vi "GetStatusGenericDrive.vi"(0 "Channel Properties":T1={"Channel Name"="", "Vel. Default"=5.0, "Acc. Default"=5.0, "Vel. Max"=5.0, "Vel. Min"=5.0, "Acc. Max"=5.0, "Acc. Min"=5.0, "Pulses/unit"=0.0, "Address"=0, "Pulse Offset"=0, "Pos Tolerance"=0.0, "Pulses/rev"=0.0, "Backlash/Eng units"=0.0, "Current Pos"=0.0, "Ch Status"=enum."Active", "Port Name"="", "Axis Transform mode"="", "Metadata Ch Name"="", "Type"=""} {"Current Pos" format="%.2f"; "Backlash/Eng units" format="%.2f"; "Pulses/rev" format="%.2f"; "Pos Tolerance" format="%.2f"; "Pulses/unit" format="%.2f"; "Acc. Min" format="%.2f"; "Acc. Max" format="%.2f"; "Vel. Min" format="%.2f"; "Vel. Max" format="%.2f"; "Acc. Default" format="%.2f"; "Vel. Default" format="%.2f"}, 2 "Limit switch valid?":bool, 3 "Stop on Trigger 3?":bool) -> (5 "Ready":bool, 6 "OK":bool, 7 "Position in Move":dbl format="%.2f", 8 "Error string":string)   [LabVIEW 2010]
uses:
  DriveProperties.ctl
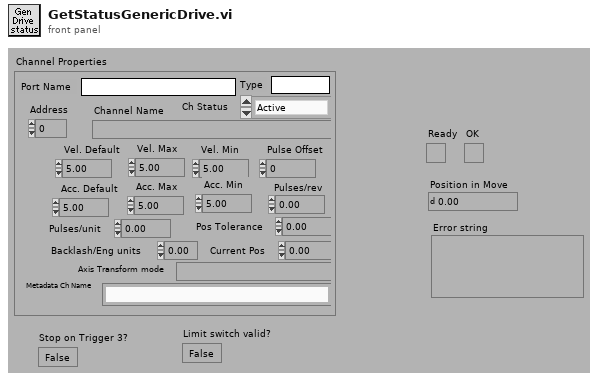
[diagram p1: front panel]
types:
  T1 = typedef "DriveProperties.ctl" = cluster{"Channel Name":string, "Vel. Default":dbl, "Acc. Default":dbl, "Vel. Max":dbl, "Vel. Min":dbl, "Acc. Max":dbl, "Acc. Min":dbl, "Pulses/unit":dbl, "Address":u8, "Pulse Offset":i32, "Pos Tolerance":dbl, "Pulses/rev":dbl, "Backlash/Eng units":dbl, "Current Pos":dbl, "Ch Status":enum16{"Active", "Offline", "Simulate"}, "Port Name":string, "Axis Transform mode":string, "Metadata Ch Name":string, "Type":string}
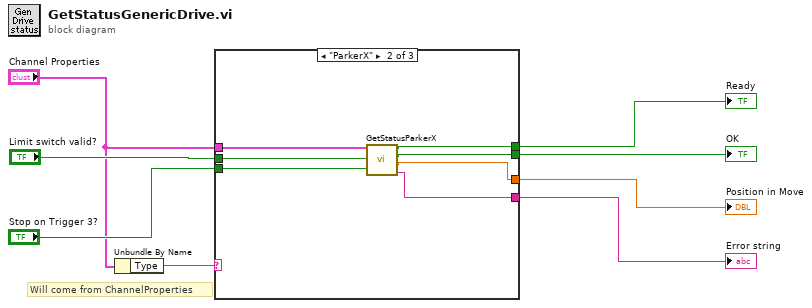
[diagram p0: block diagram]
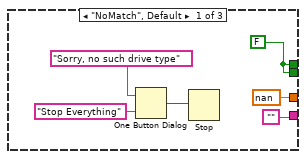
[diagram p2: hidden frame]
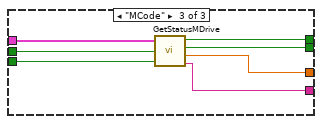
[diagram p3: hidden frame]
diagram:
  # "Will come from ChannelProperties"
  n1 = Unbundle By Name("Channel Properties") -> ("Type"=w2:string)
  n2 = case shown="\"ParkerX\"" w2 {
    tunnel: "Channel Properties" -> [_ w21 w25]
    tunnel: "Limit switch valid?" -> [_ w20 w24]
    tunnel: "Stop on Trigger 3?" -> [_ w19 w23]
    tunnel: [w14 w18 w28] -> w6
    tunnel: [w14 w17 w27] -> w5
    tunnel: [nan ("Position in Move") w16 w26] -> w4
    tunnel: ["" w15 w22] -> w3
    frame "NoMatch", Default {
      w14 = FALSE ("Good Echo")
      n3 = One Button Dialog(message="Sorry, no such drive type", button name ("OK")="Stop Everything") -> (true=w9:bool)
      n4 = Stop(stop? (T)=w9) -> ()
    }
    frame "ParkerX" {
      n5 = call "GetStatusParkerX.vi"("Channel Properties"=w21, "Limit switch valid?"=w20, "Stop on Trigger 3?"=w19) -> ("Ready"=w18:bool, "OK"=w17:bool, "Position in Move"=w16:dbl, "Error string"=w15:string)  [unwired: 2 out]
    }
    frame "MCode" {
      n6 = call "GetStatusMDrive.vi"("Channel Properties"=w25, "Limit switch valid?"=w24, "Stop on Trigger 3?"=w23) -> ("Ready"=w28:bool, "OK"=w27:bool, "Position in Move"=w26:dbl, "Error string"=w22:string)  [unwired: 2 out]
    }
  }
  "Position in Move" <- w4
  "Ready" <- w6
  "OK" <- w5
  "Error string" <- w3
